vi "EEPROMTest.vi"(8 "error in (no error)":errorcluster, 10 "method":string, 11 "Sequence Context In":refnum<k7>) -> (0 "error out":errorcluster, 2 "status":string)   [LabVIEW 2021]
uses:
  <vilib>/addons/TestStand/_TSUtility.llb/TestStand - Get Property Value (String).vi
  <vilib>/NI/JSON Support for LabVIEW/JSON Value/New JSON Value/New JSON ({Numeric}).vi
  <vilib>/NI/NI JSONRPC Server Framework/Classes/Client/Format Client Request (Auto-Increment).vi
  <vilib>/NI/JSON Support for LabVIEW/JSON Value/JSON Value.lvclass
  <vilib>/NI/NI JSONRPC Server Framework/Classes/Client/JSONRPC Client.lvclass
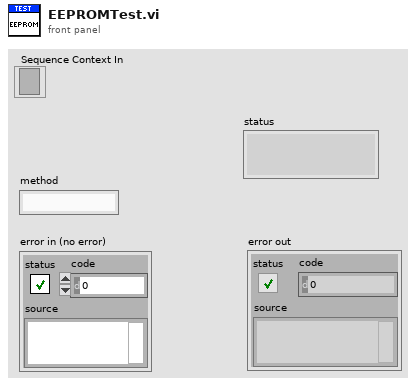
[diagram p1: front panel]
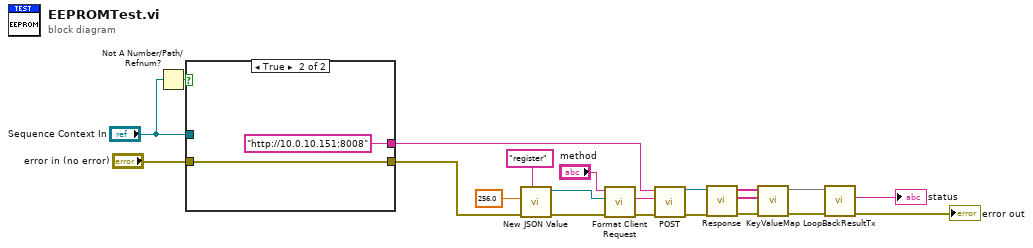
[diagram p0: block diagram]
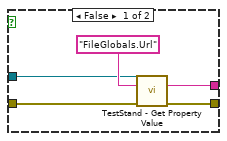
[diagram p2: hidden frame]
diagram:
  n1 = Not A Number/Path/Refnum?(number/path/refnum="Sequence Context In") -> (NaN/Path/Refnum?=w6:bool)
  n2 = case shown="True" w6 {
    tunnel: [w25 "http://10.0.10.151:8008" ("Value")] -> w21
    tunnel: [w24 w28] -> w4
    tunnel: "error in (no error)" -> [w23 w28]
    tunnel: "Sequence Context In" -> [w22 _]
    frame False {
      n3 = call-poly <vilib>:"TestStand - Get Property Value.vi"("Sequence Context In"=w22, "Lookup String"="FileGlobals.Url", "error in (no error)"=w23) -> ("Value"=w25:string, "error out"=w24:errorcluster)  [unwired: 10 in, 1 out]
    }
    frame True {
    }
  }
  n4 = call-poly <vilib>:"New JSON Value.vi"("key"="register", "error in (no error)"=w4, "value"=256.0) -> ("error out"=w5:errorcluster, "JSON Value out"=w3:refnum<class "JSON Value.lvclass">)  [unwired: 7 in]
  n5 = call-poly <vilib>:"Format Client Request.vi"("error in (no error)"=w5, "JSON Value in"=w3, "method"="method") -> ("error out"=w12:errorcluster, "Request String"=w13:string)  [unwired: 7 in]
  n6 = call "POST.vi"("error in (no error)"=w12, "Request String"=w13, "url"=w21) -> ("error out"=w14:errorcluster, "JSON Value out"=w15:refnum<class "JSON Value.lvclass">)  [unwired: 7 in]
  n7 = call "Response.vi"("error in (no error)"=w14, "JSON Value in"=w15) -> ("error out"=w16:errorcluster, "values"=w18:string[], "keys"=w17:string[])  [unwired: 7 in]
  n8 = call "KeyValueMap.vi"("error in"=w16, "values"=w18, "keys"=w17) -> ("error out"=w9:errorcluster, "map out"=w10:map{string, string})  [unwired: 7 in]
  n9 = call "LoopBackResultTx.vi"("error in (no error)"=w9, "map"=w10) -> ("error out"=→"error out":errorcluster, "status"=→"status":string)  [unwired: 8 in]
